vi "GlobalSpectHdl.vi"() -> ()   [LabVIEW 2010]
panel:
  in  "Spectrometer \nOpened":bool
  out "Spectrometer in system":bool
  in  "Spectrometer Handle":u32
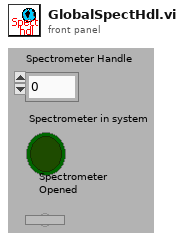
[diagram p1: front panel]
diagram:
